vi "easySAM Load_Data.vi"(9 "Load Data":bool=TRUE, 10 "Data References":T2, 11 "Data Parameters 0":T1) -> ()   [LabVIEW 2022 SP3]
uses:
  Data Record.ctl
  RF Data Value Reference.ctl
panel:
  out "Samples":i32
  out "Number Pixel Y":i32
  out "Number Pixel X":i32
  out "All A-Scans":sgl[][](graph)
  out "File":path
  out "Data Parameters":T1
  # "easySAM Data Loading Module"
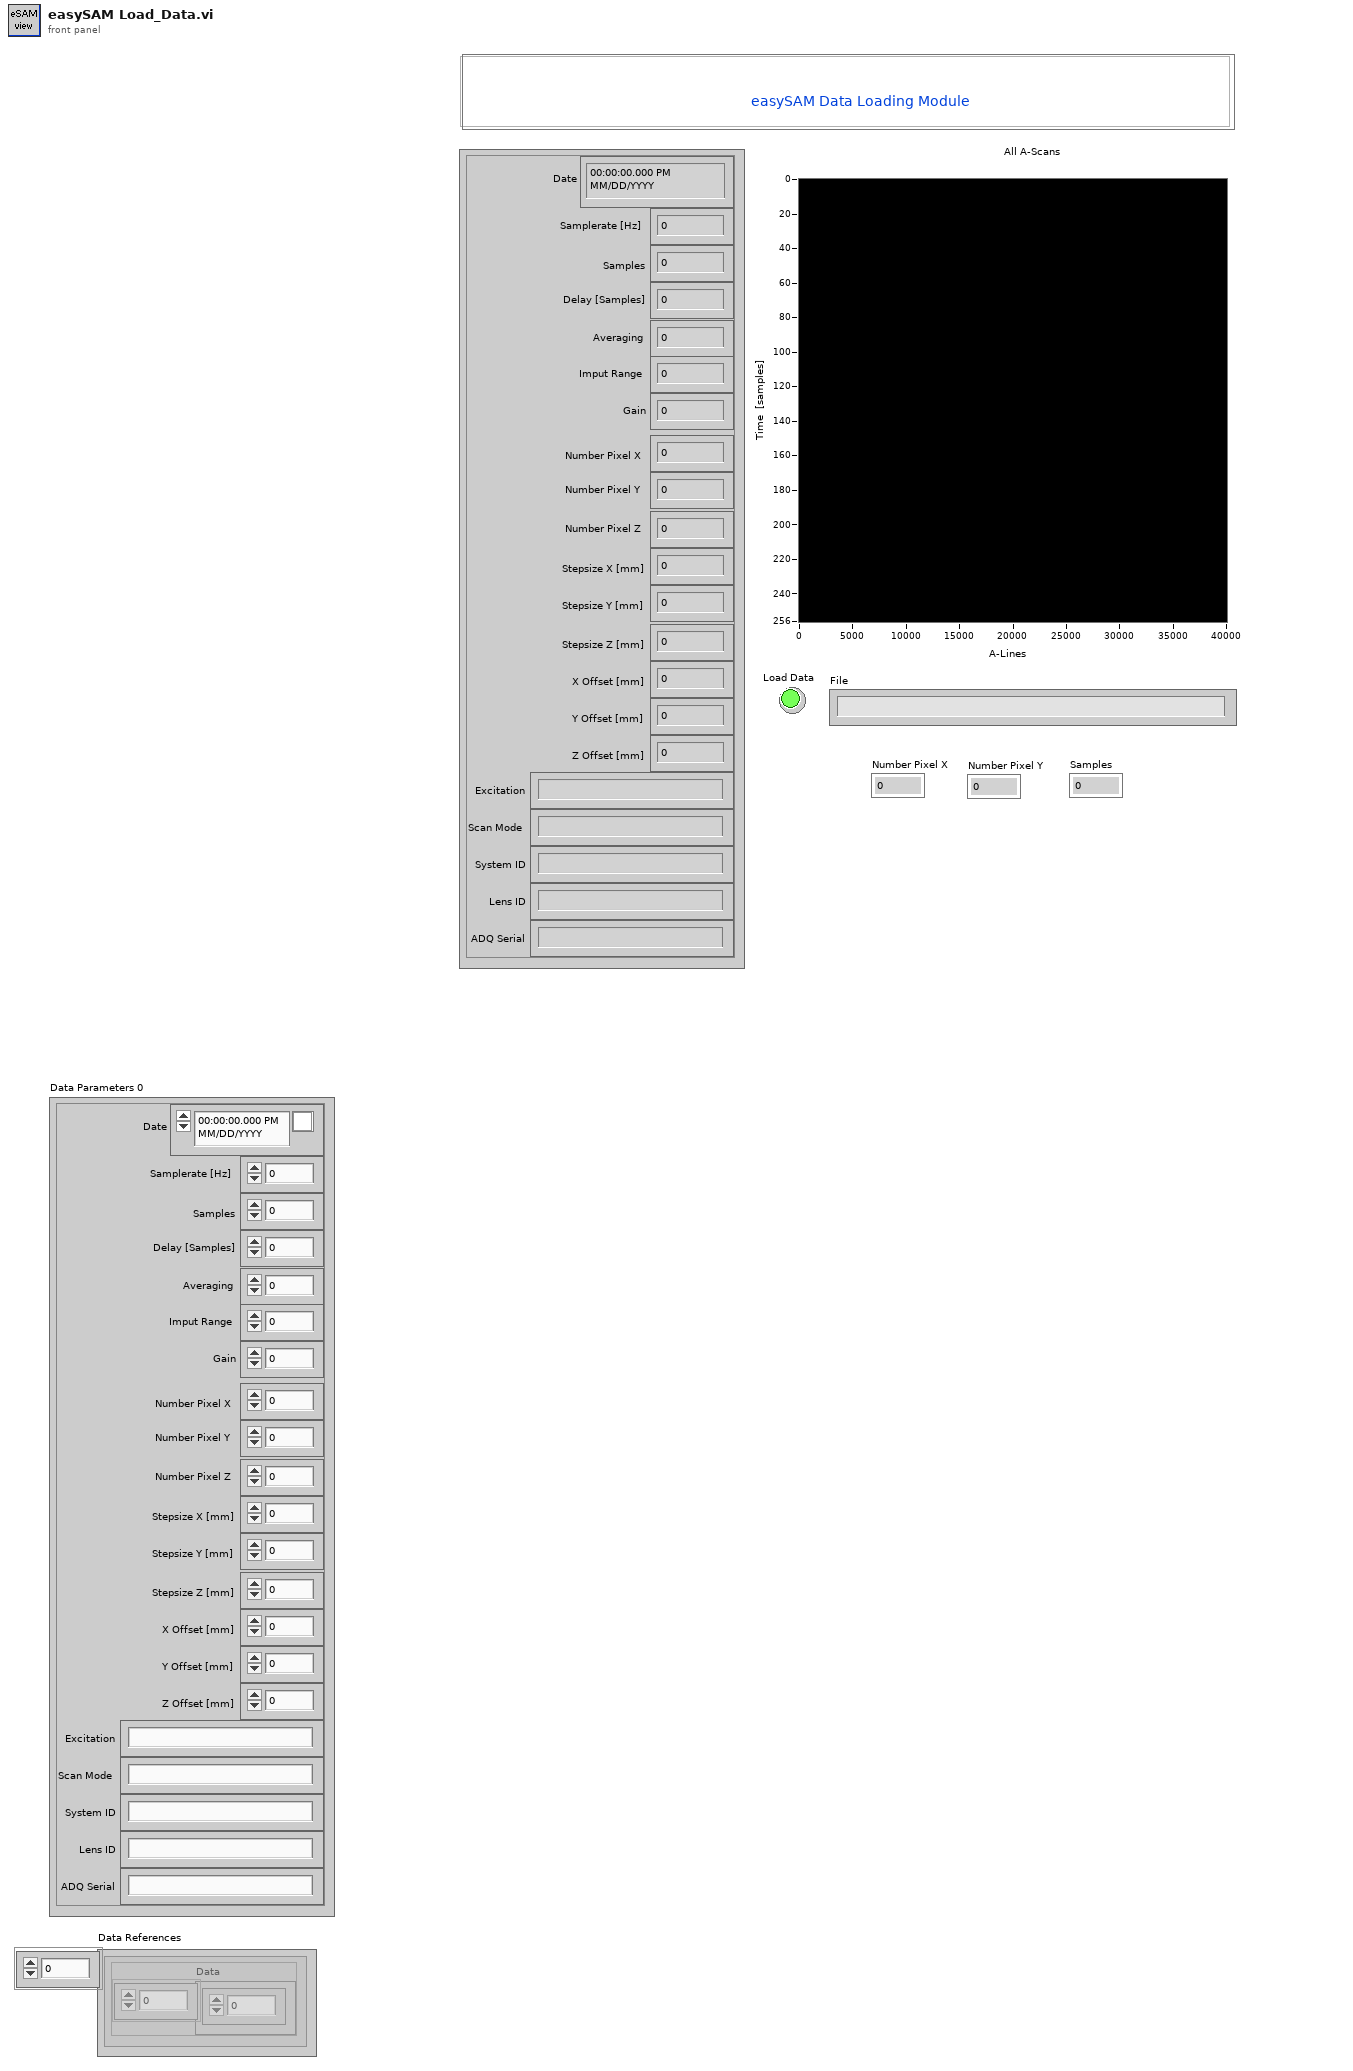
[diagram p1: front panel]
types:
  T1 = typedef "Data Record.ctl" = cluster{"Samplerate [Hz] ":dbl, "Delay [Samples]":i32, "Stepsize X [mm]":dbl, "Stepsize Y [mm]":dbl, "Z Offset [mm]":dbl, "Number Pixel X":i32, "Samples":i32, "Number Pixel Y":i32, "System ID":string, "Lens ID":string, "Date":timestamp, "X Offset [mm]":dbl, "Y Offset [mm]":dbl, "Scan Mode":string, "Excitation":string, "Gain":dbl, "Imput Range":dbl, "Averaging":i32, "ADQ Serial":string, "Stepsize Z [mm]":dbl, "Number Pixel Z":i32}
  T2 = typedef "RF Data Value Reference.ctl" = cluster{"Data":sgl[]}[]
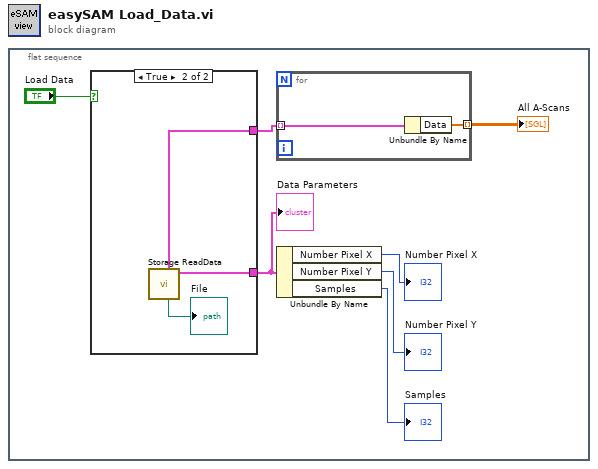
[diagram p0: block diagram]
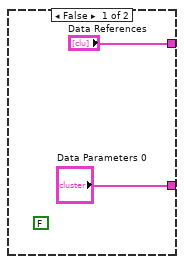
[diagram p2: hidden frame]
diagram:
  n1 = flat-sequence {
    frame #0 {
      n2 = case shown="True" "Load Data" {
        tunnel: ["Data Parameters 0" w11] -> w7
        tunnel: ["Data References" w12] -> w6
        frame False {
          (unwired) FALSE ("cancelled")
        }
        frame True {
          n3 = call "Storage ReadData.vi"() -> ("Acoustic Data"=w11:T1, "path"=→"File":path, "Data Referenzen"=w12:T2)  [unwired: 6 in, 3 out]
        }
      }
      "Data Parameters" <- w7
      n4 = for {
        tunnel: w6 -> [w14] mode=indexing
        tunnel: [w13] -> w5 mode=indexing
        n5 = Unbundle By Name(w14) -> ("Data"=w13:sgl[])
      }
      "All A-Scans" <- w5
      n6 = Unbundle By Name(w7) -> ("Number Pixel X"=→"Number Pixel X":i32, "Number Pixel Y"=→"Number Pixel Y":i32, "Samples"=→"Samples":i32)
    }
  }
